vi "LIA Read DMAs.vi"(8 "error in":errorcluster, 9 "DMA?":bool, 10 "Number of Elements":u32, 11 "FPGA VI Reference In":refnum<k20>) -> (0 "error out":errorcluster, 1 "Numeric":fxp<+/-,49,1>, 2 "Elements Remaining":u32, 3 "FPGA VI Reference Out":refnum<k20>, 5 "VCO":sgl[](array[numeric]), 7 "AI":sgl[](array[numeric]))   [LabVIEW 2017]
uses:
  Program Files (x86)/National Instruments/LabVIEW 2017/examples/Lock-In Amplifier/lib/host/Public/fpga type.ctl
  <vilib>/Utility/error.llb/Error Cluster From Error Code.vi
  <vilib>/rvi/errors/niLvFpgaAdjustHostInterfaceError.vi
  <vilib>/rvi/interface/nirviReadWriteControl/nirviReadWriteControl.xnode
  <vilib>/rvi/interface/nirviMethod/nirviMethod.xnode
  Program Files (x86)/National Instruments/LabVIEW 2017/examples/Lock-In Amplifier/lib/host/Lock-In Amplifier Example Host.lvlib
  <vilib>/FPGAPlugInAG/Dynamic/niLvFpga_ReadFifo_Dynamic.vi
  <vilib>/rvi/errors/niLvFpgaMergeErrorWithErrorCode.vi
  NiFpgaLv.dll
  <vilib>/rvi/interface/Simulation/niFpgaSimulationCallBeginRW.vi
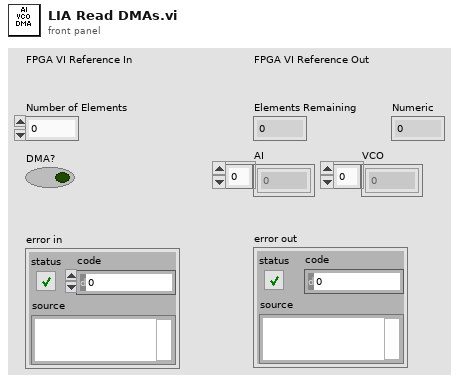
[diagram p1: front panel]
types:
  T1 = typedef "Lock-In Amplifier Example Host.lvlib/fpga type.ctl" = refnum<k20>
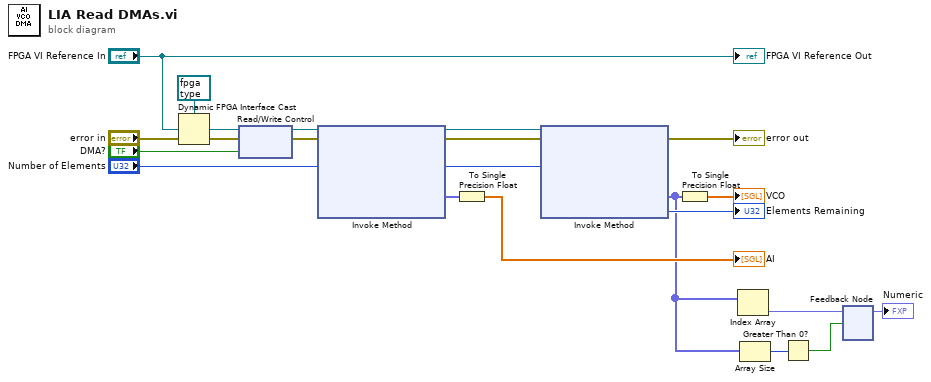
[diagram p0: block diagram]
diagram:
  n1 = Dynamic FPGA Interface Cast(Session In=T1 refnum ("fpga type"), Type="FPGA VI Reference In") -> (Session Out=w8:T1)
  n2 = xnode "Read/Write Control"("FPGA VI Reference In"=w8, "error in"="error in", "DMA?"="DMA?") -> ("FPGA VI Reference Out"=w7:T1, "error out"=w9:errorcluster)
  n3 = xnode "Invoke Method"("FPGA VI Reference In"=w7, "error in"=w9, "Number of Elements"="Number of Elements") -> ("FPGA VI Reference Out"=w17:T1, "error out"=w16:errorcluster, "Data"=w14:fxp<+/-,18,1>[])  [unwired: 1 in, 1 out]
  n4 = To Single Precision Float(number=w14) -> (single precision float=→"AI":sgl[])
  n5 = xnode "Invoke Method"("FPGA VI Reference In"=w17, "error in"=w16, "Number of Elements"="Number of Elements") -> ("error out"=→"error out":errorcluster, "Data"=w5:fxp<+/-,49,1>[], "Elements Remaining"=→"Elements Remaining":u32)  [unwired: 1 in, 1 out]
  n6 = To Single Precision Float(number=w5) -> (single precision float=→"VCO":sgl[])
  n7 = Index Array(array=w5) -> (element=w3:fxp<+/-,49,1>)  [unwired: 1 in]
  n8 = Array Size(array=w5) -> (size(s)=w4:i32)
  n9 = Greater Than 0?(x=w4) -> (x > 0?=w2:bool)
  n10 = feedback-in #1(w3, w2) -> ()
  n11 = feedback #1() -> (→"Numeric":fxp<+/-,49,1>)  [unwired: 1 in]
  "FPGA VI Reference Out" <- "FPGA VI Reference In"
